vi "Status Word Monitor - Fault Troubleshooting.vi"() -> ()   [LabVIEW 2014]
panel:
  in  "Clear Errors":bool
  in  "Manual Control Word":u16
  in  "Manual Control Word":bool
  in  "Send 0 Command":bool
  out "error out":errorcluster
  out "Status Word":u16
  in  "stop":bool
  out "Status History":u16[](array[numeric])
  # "1) Run VI\n2) Drive Should Enable Automatically\n\n3) Force a Drive Fault\n\n4) Click NI Enable Sequence\n5) See that drive moves out of fault state\nWithout us ever sending Fault Reset Command"
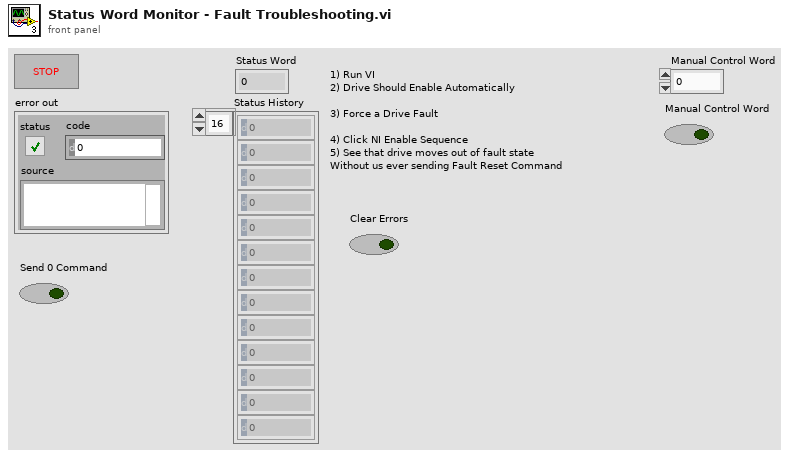
[diagram p1: front panel]
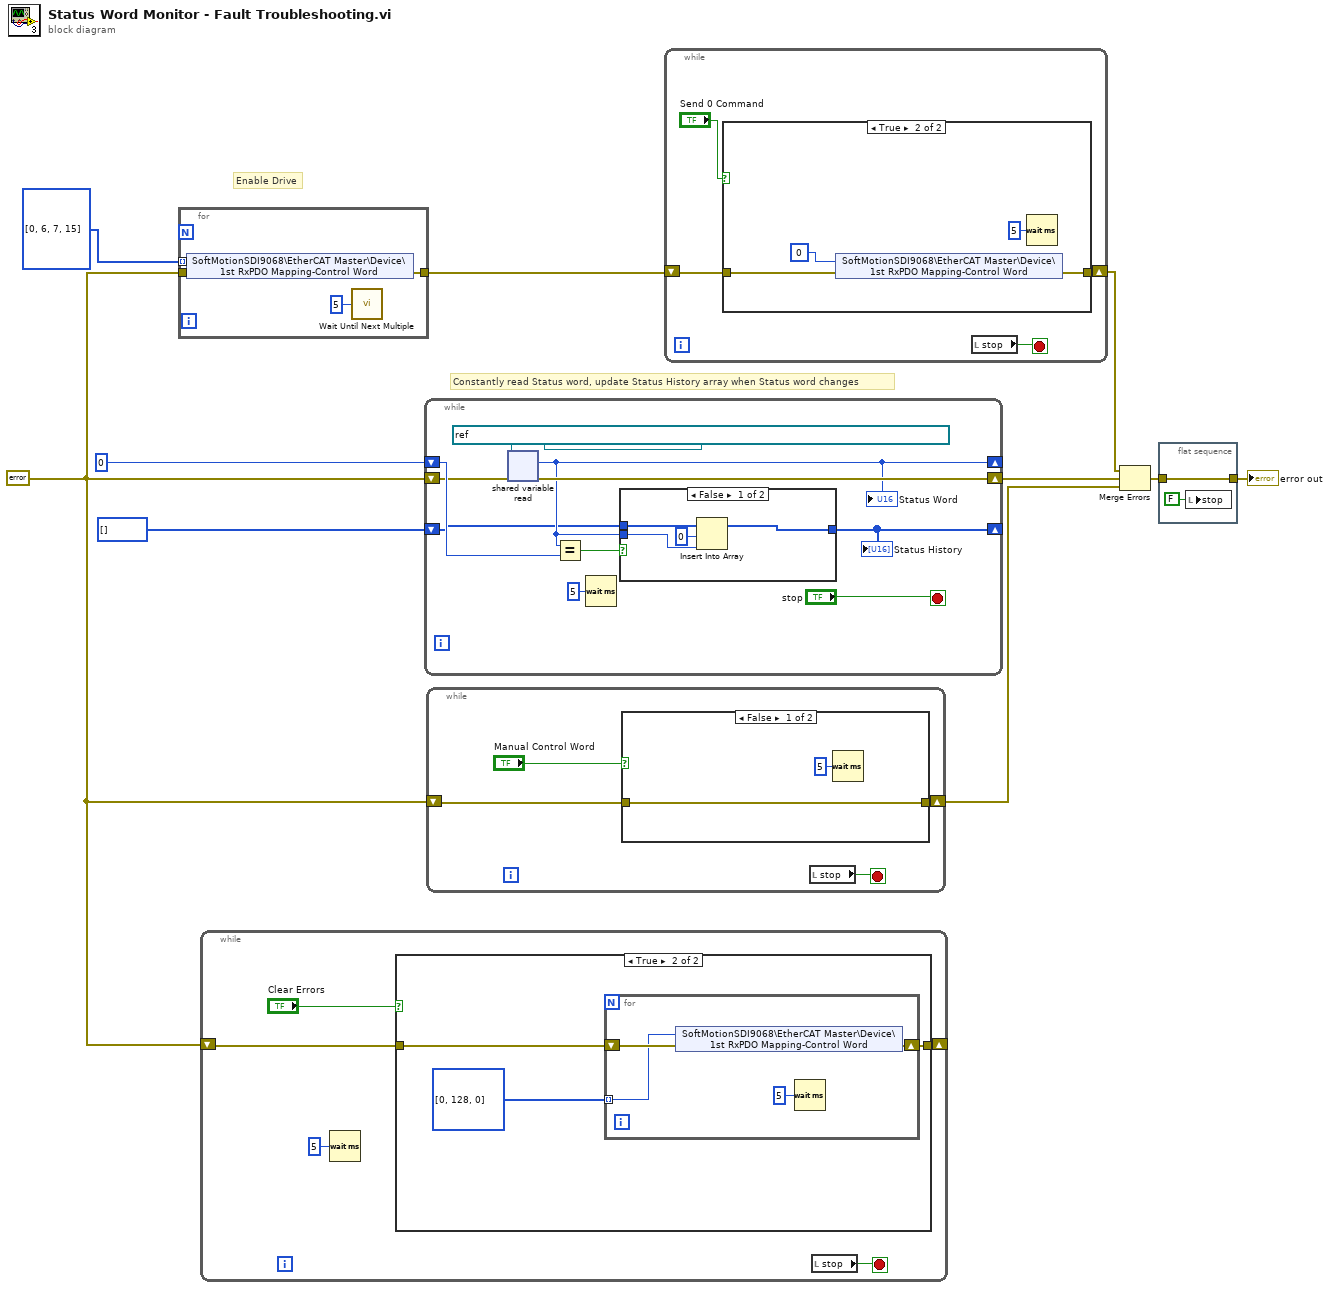
[diagram p0: block diagram]
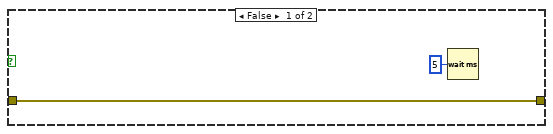
[diagram p2: hidden frame]
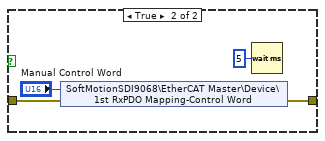
[diagram p3: hidden frame]
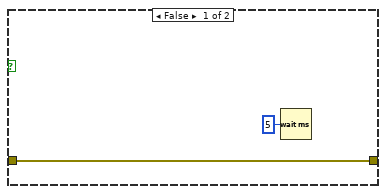
[diagram p4: hidden frame]
diagram:
  w1 = errorcluster {"status"=FALSE, "code"=0, "source"=""} ("error IO")
  # "Constantly read Status word, update Status History array when Status word changes"
  # "Enable Drive"
  n1 = for {
    tunnel: u16[] [0, 6, 7, 15] -> [w14] mode=indexing
    tunnel: [w12] -> w6
    tunnel: w1 -> [w11]
    n2 = shared-variable "SoftMotionSDI9068\\EtherCAT Master\\Device\\1st RxPDO Mapping-Control Word"(w14, error in=w11) -> (error out=w12:errorcluster)
    n3 = call "Wait Until Next Multiple"("Count(mSec)"=u32 5) -> ()  [unwired: 1 out]
  }
  n4 = while {
    shift-right: [w16] -> _
    shift-left: w1 -> [w19]
    stop <- w18 stop-if-true
    n5 = Wait (ms)(milliseconds to wait=u32 5) -> ()  [unwired: 1 out]
    n6 = case shown="True" "Clear Errors" {
      tunnel: w19 -> [w20 w24]
      tunnel: [w20 w23] -> w16
      frame False {
        n7 = Wait (ms)(milliseconds to wait=u32 5) -> ()  [unwired: 1 out]
      }
      frame True {
        n8 = for {
          shift-right: [w27] -> w23
          shift-left: w24 -> [w28]
          tunnel: u16[] [0, 128, 0] -> [w26] mode=indexing
          n9 = shared-variable "SoftMotionSDI9068\\EtherCAT Master\\Device\\1st RxPDO Mapping-Control Word"(w26, error in=w28) -> (error out=w27:errorcluster)
          n10 = Wait (ms)(milliseconds to wait=u32 5) -> ()  [unwired: 1 out]
        }
      }
    }
    n11 = local read "stop"() -> (w18:bool)
  }
  n12 = while {
    shift-right: [w32] -> _
    shift-left: u16 0 -> [w37]
    shift-right: [w34] -> w7
    shift-left: w1 -> [w35]
    shift-right: [w31] -> _
    shift-left: u16[] [] -> [w30]
    stop <- "stop" stop-if-true
    n13 = shared-variable-read(refnum<k21> "ni.var.io://SoftMotionSDI9068/EtherCAT Master/Device/1st TxPDO Mapping-Status Word" ("shared variable refnum in"), w35) -> (w34:errorcluster, w32:u16)  [unwired: 1 out]
    "Status Word" <- w32
    n14 = Equal?(x=w32, y=w37) -> (x = y?=w33:bool)
    n15 = Wait (ms)(milliseconds to wait=u32 5) -> ()  [unwired: 1 out]
    n16 = case shown="False" w33 {
      tunnel: w32 -> [w41 _]
      tunnel: [w40 w43] -> w31
      tunnel: w30 -> [w42 w43]
      frame False {
        n17 = Insert Into Array(array=w42, index=0, new element=w41) -> (w40:u16[])
      }
      frame True {
      }
    }
    "Status History" <- w31
  }
  n18 = while {
    shift-right: [w44] -> w4
    shift-left: w1 -> [w47]
    stop <- w46 stop-if-true
    n19 = case shown="False" "Manual Control Word" {
      tunnel: w47 -> [w48 w53]
      tunnel: [w48 w52] -> w44
      frame False {
        n20 = Wait (ms)(milliseconds to wait=u32 5) -> ()  [unwired: 1 out]
      }
      frame True {
        n21 = shared-variable "SoftMotionSDI9068\\EtherCAT Master\\Device\\1st RxPDO Mapping-Control Word"("Manual Control Word", error in=w53) -> (error out=w52:errorcluster)
        n22 = Wait (ms)(milliseconds to wait=u32 5) -> ()  [unwired: 1 out]
      }
    }
    n23 = local read "stop"() -> (w46:bool)
  }
  n24 = while {
    shift-right: [w54] -> w5
    shift-left: w6 -> [w57]
    stop <- w56 stop-if-true
    n25 = case shown="True" "Send 0 Command" {
      tunnel: w57 -> [w58 w63]
      tunnel: [w58 w62] -> w54
      frame False {
        n26 = Wait (ms)(milliseconds to wait=u32 5) -> ()  [unwired: 1 out]
      }
      frame True {
        n27 = shared-variable "SoftMotionSDI9068\\EtherCAT Master\\Device\\1st RxPDO Mapping-Control Word"(u16 0, error in=w63) -> (error out=w62:errorcluster)
        n28 = Wait (ms)(milliseconds to wait=u32 5) -> ()  [unwired: 1 out]
      }
    }
    n29 = local read "stop"() -> (w56:bool)
  }
  n30 = Merge Errors(w5, w7, w4) -> (w2:errorcluster)
  n31 = flat-sequence {
    tunnel: [w65] -> w3
    tunnel: w2 -> [w65]
    frame #0 {
      n32 = local write "stop"(FALSE ("stop")) -> ()
    }
  }
  "error out" <- w3
